vi "Process PMU Configuration.vi"(8 "error in (no error)":errorcluster, 10 "PMU Configuration":T1(array[cluster]), 11 "Phasor Data Concentrator in":refnum<class "Phasor Data Concentrator.lvclass">) -> (0 "error out":errorcluster, 3 "Phasor Data Concentrator out":refnum<class "Phasor Data Concentrator.lvclass">)   [LabVIEW 2013, in "PMU Recorder Light.lvlib" / "Phasor Data Concentrator.lvclass"]
uses:
  Phasor Data Concentrator.lvclass
  Phasor Data Concentrator.lvclass/Phasor Data Concentrator.ctl
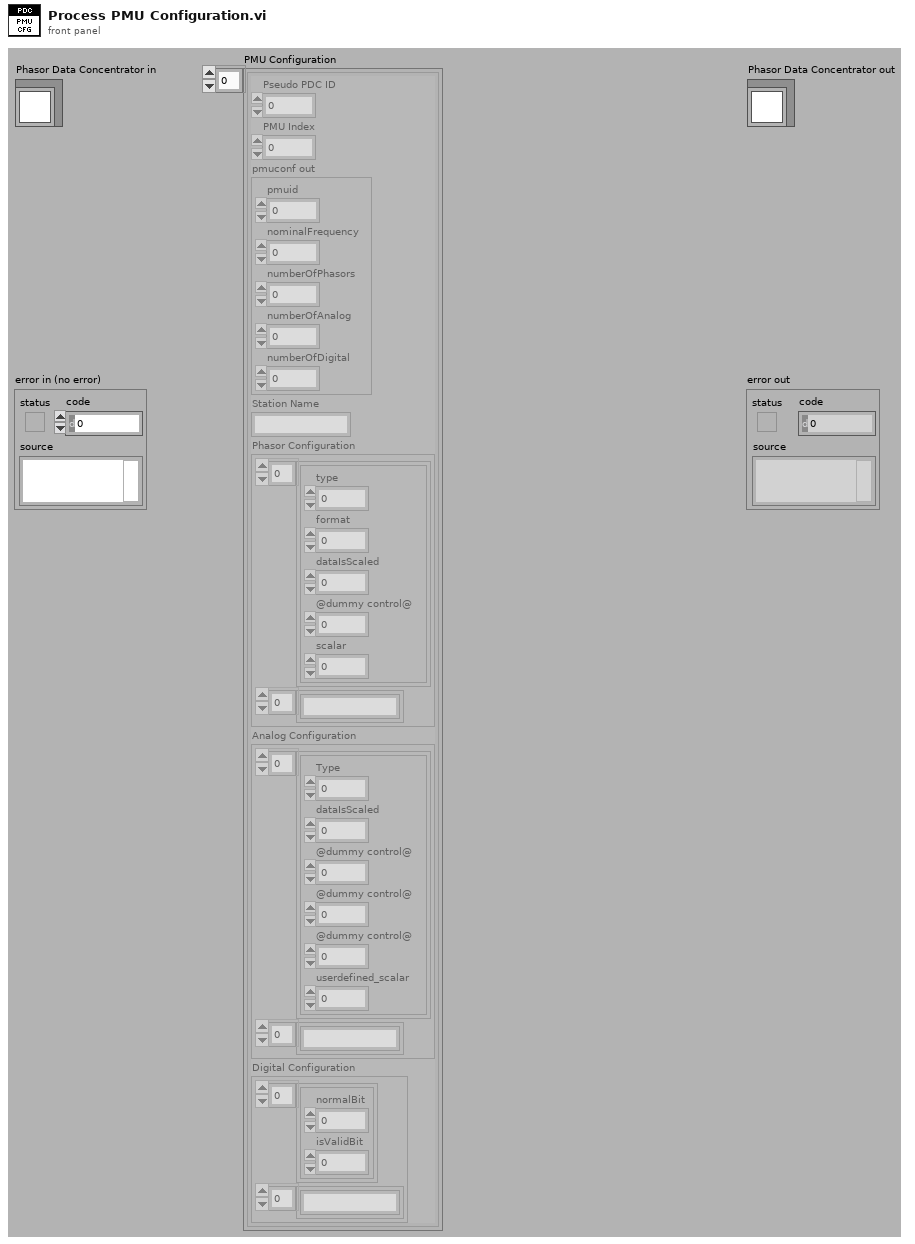
[diagram p1: front panel]
types:
  T1 = cluster{"Pseudo PDC ID":i32, "PMU Index":i32, "pmuconf out":cluster{"pmuid":i32, "nominalFrequency":sgl, "numberOfPhasors":i32, "numberOfAnalog":i32, "numberOfDigital":i32}, "Station Name":string, "Phasor Configuration":cluster{cluster{"type":u8, "format":u8, "dataIsScaled":u8, "@dummy control@":i8, "scalar":sgl}[], string[]}, "Analog Configuration":cluster{cluster{"Type":i32, "dataIsScaled":u8, "@dummy control@":i8, "@dummy control@":i8, "@dummy control@":i8, "userdefined_scalar":sgl}[], string[]}, "Digital Configuration":cluster{cluster{"normalBit":u8, "isValidBit":u8}[], string[]}}[]
  T2 = cluster{"Main ":cluster{"PMU ID Code":i32, "PMU Name":string, "Nominal Frequency":sgl, "Number of Phasors":i32, "Number of Analog":i32, "Number of Digital":i32}, "Phasor Configuration":cluster{"Name":string, "Type":u8, "Format":u8, "Data Is Scaled":u8, "Scalar":sgl}[], "Analog Configuration":cluster{"Name":string, "Type":i32, "Data Is Scaled":u8, "User Defined Scalar":sgl}[], "Digital Configuration":cluster{"Name":string, "Normal Bit":u8, "Is Valid Bit":u8}[]}
  T3 = cluster{"PMU ID Code":i32, "PMU Name":string, "Nominal Frequency":sgl, "Number of Phasors":i32, "Number of Analog":i32, "Number of Digital":i32}
  T4 = cluster{cluster{"type":u8, "format":u8, "dataIsScaled":u8, "@dummy control@":i8, "scalar":sgl}[], string[]}
  T5 = cluster{cluster{"Type":i32, "dataIsScaled":u8, "@dummy control@":i8, "@dummy control@":i8, "@dummy control@":i8, "userdefined_scalar":sgl}[], string[]}
  T6 = cluster{cluster{"normalBit":u8, "isValidBit":u8}[], string[]}
  T7 = cluster{"pmuid":i32, "nominalFrequency":sgl, "numberOfPhasors":i32, "numberOfAnalog":i32, "numberOfDigital":i32}
  T8 = cluster{"Name":string, "Type":u8, "Format":u8, "Data Is Scaled":u8, "Scalar":sgl}[]
  T9 = cluster{"Name":string, "Type":i32, "Data Is Scaled":u8, "User Defined Scalar":sgl}[]
  T10 = cluster{"Name":string, "Normal Bit":u8, "Is Valid Bit":u8}[]
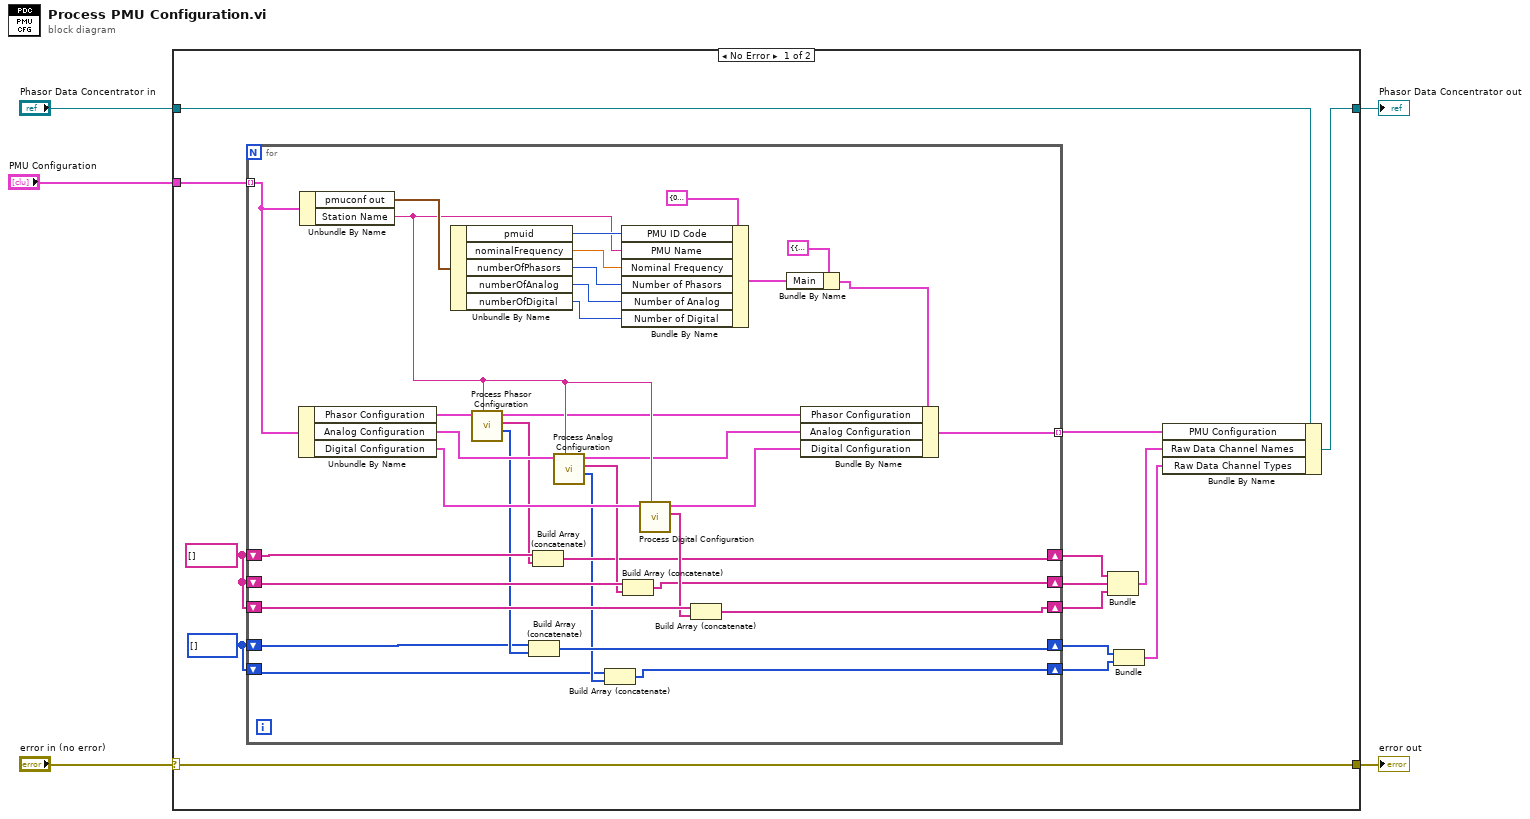
[diagram p0: block diagram]
diagram:
  n1 = case shown="No Error" "error in (no error)" {
    selector: "error in (no error)" -> [w19 w55]
    tunnel: [w19 w55] -> w4
    tunnel: [w17 w54] -> w2
    tunnel: "Phasor Data Concentrator in" -> [w18 w54]
    tunnel: "PMU Configuration" -> [w16 _]
    frame No Error {
      w9 = u8[] []
      w15 = string[] []
      n2 = for {
        tunnel: w16 -> [w45] mode=indexing
        shift-right: [w27] -> w12
        shift-left: w15 -> [w35]
        shift-right: [w28] -> w13
        shift-left: w15 -> [w33]
        shift-right: [w29] -> w11
        shift-left: w15 -> [w31]
        tunnel: [w26] -> w14 mode=indexing
        shift-right: [w23] -> w8
        shift-left: w9 -> [w24]
        shift-right: [w20] -> w7
        shift-left: w9 -> [w21]
        n3 = Unbundle By Name(w45) -> ("Phasor Configuration"=w44:T4, "Analog Configuration"=w43:T5, "Digital Configuration"=w42:T6)
        n4 = Unbundle By Name(w45) -> ("pmuconf out"=w52:T7, "Station Name"=w41:string)
        n5 = Unbundle By Name(w52) -> ("pmuid"=w51:i32, "nominalFrequency"=w50:sgl, "numberOfPhasors"=w49:i32, "numberOfAnalog"=w48:i32, "numberOfDigital"=w47:i32)
        n6 = call "Process Phasor Configuration.vi"("PMU Name"=w41, "Phasor Configuration In"=w44) -> ("Phasor Types"=w25:u8[], "Phasor Channel Names"=w34:string[], "Phasor Configuration Out"=w38:T8)  [unwired: 7 in]
        n7 = Build Array (concatenate)(w24, w25) -> (w23:u8[])
        n8 = Build Array (concatenate)(w35, w34) -> (w27:string[])
        n9 = call "Process Analog Configuration.vi"("PMU Name"=w41, "Analog Configuration In"=w43) -> ("Analog Channel Types"=w22:u8[], "Analog Channel Names"=w32:string[], "Analog Configuration Out"=w37:T9)  [unwired: 7 in]
        n10 = Build Array (concatenate)(w21, w22) -> (w20:u8[])
        n11 = Bundle By Name(cluster=T3 {"PMU ID Code"=0, "PMU Name"="", "Nominal Frequency"=0.0, "Number of Phasors"=0, "Number of Analog"=0, "Number of Digital"=0} ("Main"), "PMU ID Code"=w51, "PMU Name"=w41, "Nominal Frequency"=w50, "Number of Phasors"=w49, "Number of Analog"=w48, "Number of Digital"=w47) -> (w46:T3)
        n12 = Build Array (concatenate)(w33, w32) -> (w28:string[])
        n13 = call "Process Digital Configuration.vi"("PMU Name"=w41, "Digital Configuration In"=w42) -> ("Digital Channel Names"=w30:string[], "Digital Configuration Out"=w36:T10)  [unwired: 8 in]
        n14 = Build Array (concatenate)(w31, w30) -> (w29:string[])
        n15 = Bundle By Name(cluster=T2 {"Main "={"PMU ID Code"=0, "PMU Name"="", "Nominal Frequency"=0.0, "Number of Phasors"=0, "Number of Analog"=0, "Number of Digital"=0}, "Phasor Configuration"=[], "Analog Configuration"=[], "Digital Configuration"=[]} ("PMU Configuration"), "Main"=w46) -> (w39:T2)
        n16 = Bundle By Name(cluster=w39, "Phasor Configuration"=w38, "Analog Configuration"=w37, "Digital Configuration"=w36) -> (w26:T2)
      }
      n17 = Bundle(w12, w13, w11) -> (w10:cluster{string[], string[], string[]})  [unwired: 1 in]
      n18 = Bundle(w8, w7) -> (w6:cluster{u8[], u8[]})  [unwired: 1 in]
      n19 = Bundle By Name(cluster=w18, "PMU Configuration"=w14, "Raw Data Channel Names"=w10, "Raw Data Channel Types"=w6) -> (w17:refnum<class "Phasor Data Concentrator.lvclass">)
    }
    frame Error {
    }
  }
  "error out" <- w4
  "Phasor Data Concentrator out" <- w2
